vi "USB2XXX_PowerAnalyzer_Test.vi"() -> ()   [LabVIEW 2010]
panel:
  in  "FilterLevel":i32=500
  in  "UseZeroSet":u8=1
  in  "AutoZeroSet":u8
  out "功率":dbl[](graph)=[0.0, 0.0, 0.0, 0.0, 0.0, 0.0, 1.7578661454081409e-07, 0.0, 0.0, 0.0, 0.0, 0.0, 0.0, 0.0, 0.0, 0.0, 0.0, 0.0, 0.0, 0.0, 0.0, 0.0, 0.0, 1.7578661454081409e-07, 0.0, 1.7578661454081409e-07, 0.0, 0.0, 0.0, 0.0]
  out "电压":dbl[](graph)
  out "电流":dbl[](graph)=[0.0, 0.0, 0.0, 0.0, 0.0, 0.0009375143053330281, 0.0, 0.0, 0.0, 0.0, 0.0, 0.0, 0.0009375143053330281, 0.0009375143053330281, 0.0009375143053330281, 0.0, 0.0, 0.0009375143053330281, 0.0009375143053330281, 0.0, 0.0, 0.0, 0.0009375143053330281, 0.0, 0.0, 0.0009375143053330281, 0.0009375143053330281, 0.0, 0.0, 0.0]
  in  "stop":bool
  in  "SamplingRate":i32=1000
  in  "Device Index":i32(ring) items=["0", "1", "2", "3", "4", "5"]
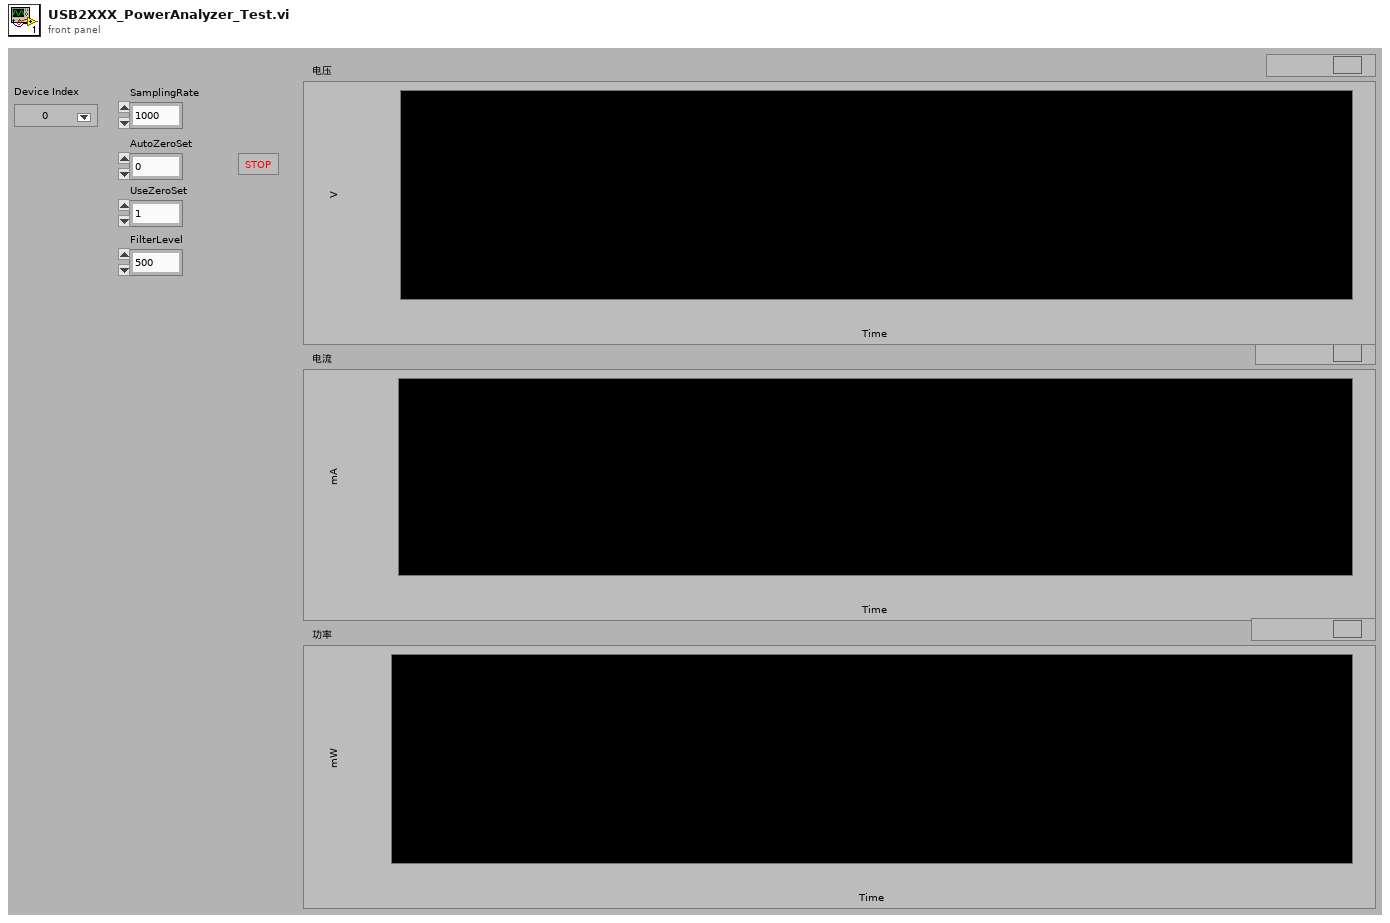
[diagram p1: front panel]
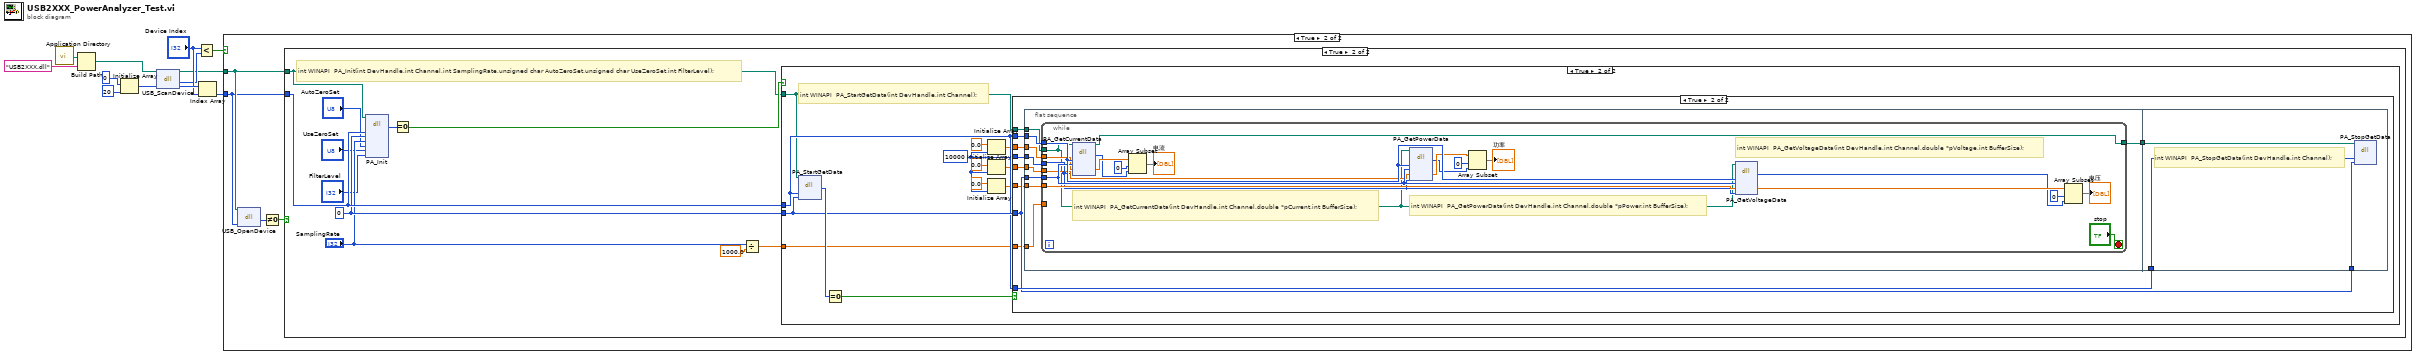
[diagram p0: block diagram]
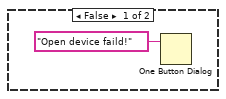
[diagram p3: hidden frame]
diagram:
  n1 = call <vilib>:"Application Directory.vi"() -> ("Application Directory"=w2:path)
  n2 = Build Path(base path=w2, name or relative path="USB2XXX.dll") -> (appended path=w1:path)
  n3 = Initialize Array(0, 20 ("dimension size")) -> (w9:i32[])
  n4 = dll-call lib="E:/OtherWork/STM32/USB2XXX_Example/trunk/Labview/PublicFiles/USB2XXX.dll" fn="USB_ScanDevice"(path in=w1, "pDevNum"=w9) -> (path out=w5:path, "return type"=w7:i32, "pDevNum"=w12:i32[])  [unwired: 2 in, 1 out]
  n5 = Less?(x="Device Index", y=w7) -> (x < y?=w6:bool)
  n6 = Index Array(array=w12, index="Device Index") -> (element=w4:i32)
  n7 = case shown="True" w6 {
    tunnel: w5 -> [_ w14]
    tunnel: w4 -> [_ w13]
    frame False {
    }
    frame True {
      n8 = dll-call lib="E:/OtherWork/STM32/USB2XXX_Example/trunk/Labview/PublicFiles/USB2XXX.dll" fn="USB_OpenDevice"(path in=w14, "DevIndex"=w13) -> ("return type"=w16:u8)  [unwired: 3 in, 2 out]
      n9 = Not Equal To 0?(x=w16) -> (x != 0?=w15:bool)
      n10 = case shown="True" w15 {
        tunnel: w13 -> [_ w24]
        tunnel: w14 -> [_ w25]
        frame False {
          n11 = One Button Dialog(message="Open device faild!") -> ()  [unwired: 1 in, 1 out]
        }
        frame True {
          w23 = 0 ("Channel")
          # "int WINAPI  PA_Init(int DevHandle,int Channel,int SamplingRate,unsigned char AutoZeroSet,unsigned char UseZeroSet,int FilterLevel);"
          n12 = dll-call lib="E:/Projects/USB2XXX/trunk/USB2XXX/USB2XXX/vs2010/Release/USB2XXX.*" fn="PA_Init"(path in=w25, "DevHandle"=w24, "Channel"=w23, "SamplingRate"="SamplingRate", "AutoZeroSet"="AutoZeroSet", "UseZeroSet"="UseZeroSet", "FilterLevel"="FilterLevel") -> ("return type"=w18:i32)  [unwired: 8 in, 2 out]
          n13 = Equal To 0?(x=w18) -> (x = 0?=w28:bool)
          n14 = Divide(x="SamplingRate", y=1000.0 ("element")) -> (x/y=w26:dbl)
          n15 = case shown="True" w28 {
            tunnel: w24 -> [_ w38]
            tunnel: w23 -> [_ w39]
            tunnel: w26 -> [_ w30]
            tunnel: w25 -> [_ w29]
            frame False {
            }
            frame True {
              w31 = 10000 ("dimension size")
              # "int WINAPI  PA_StartGetData(int DevHandle,int Channel);"
              n16 = dll-call lib="E:/Projects/USB2XXX/trunk/USB2XXX/USB2XXX/vs2010/Release/USB2XXX.*" fn="PA_StartGetData"(path in=w29, "DevHandle"=w38, "Channel"=w39) -> ("return type"=w41:i32)  [unwired: 4 in, 2 out]
              n17 = Equal To 0?(x=w41) -> (x = 0?=w40:bool)
              n18 = Initialize Array(0.0 ("element"), w31) -> (w34:dbl[])
              n19 = Initialize Array(0.0 ("element"), w31) -> (w33:dbl[])
              n20 = Initialize Array(0.0 ("element"), w31) -> (w32:dbl[])
              n21 = case shown="True" w40 {
                tunnel: w38 -> [_ w51]
                tunnel: w39 -> [_ w49]
                tunnel: w38 -> [_ w50]
                tunnel: w34 -> [_ w48]
                tunnel: w33 -> [_ w47]
                tunnel: w32 -> [_ w46]
                tunnel: w31 -> [_ w45]
                tunnel: w30 -> [_ w44]
                tunnel: w29 -> [_ w43]
                frame False {
                }
                frame True {
                  n22 = flat-sequence {
                    tunnel: w50 -> [w60]
                    tunnel: w49 -> [w59]
                    tunnel: w48 -> [w58]
                    tunnel: w47 -> [w57]
                    tunnel: w46 -> [w56]
                    tunnel: w45 -> [w55]
                    tunnel: w44 -> [w54]
                    tunnel: w43 -> [w53]
                    tunnel: [w52] -> w42
                    tunnel: w51 -> [w84]
                    tunnel: w49 -> [w83]
                    tunnel: w42 -> [w82]
                    frame #0 {
                      n23 = while {
                        tunnel: w60 -> [w80]
                        tunnel: w59 -> [w79]
                        tunnel: w58 -> [w78]
                        tunnel: w57 -> [w77]
                        tunnel: w56 -> [w76]
                        tunnel: w55 -> [w75]
                        tunnel: w54 -> [_]
                        tunnel: w53 -> [w65]
                        tunnel: [w64] -> w52
                        stop <- "stop" stop-if-true
                        # "int WINAPI  PA_GetVoltageData(int DevHandle,int Channel,double *pVoltage,int BufferSize);"
                        # "int WINAPI  PA_GetPowerData(int DevHandle,int Channel,double *pPower,int BufferSize);"
                        # "int WINAPI  PA_GetCurrentData(int DevHandle,int Channel,double *pCurrent,int BufferSize);"
                        n24 = dll-call lib="E:/Projects/USB2XXX/trunk/USB2XXX/USB2XXX/vs2010/Release/USB2XXX.*" fn="PA_GetCurrentData"(path in=w65, "DevHandle"=w80, "Channel"=w79, "pCurrent"=w78, "BufferSize"=w75) -> (path out=w64:path, "return type"=w72:i32, "pCurrent"=w74:dbl[])  [unwired: 5 in, 1 out]
                        n25 = Array Subset(array=w74, index=0, length=w72) -> (→"电流":dbl[])
                        n26 = dll-call lib="E:/Projects/USB2XXX/trunk/USB2XXX/USB2XXX/vs2010/Release/USB2XXX.*" fn="PA_GetPowerData"(path in=w65, "DevHandle"=w80, "Channel"=w79, "pPower"=w77, "BufferSize"=w75) -> ("return type"=w66:i32, "pPower"=w69:dbl[])  [unwired: 5 in, 2 out]
                        n27 = Array Subset(array=w69, index=0, length=w66) -> (→"功率":dbl[])
                        n28 = dll-call lib="E:/Projects/USB2XXX/trunk/USB2XXX/USB2XXX/vs2010/Release/USB2XXX.*" fn="PA_GetVoltageData"(path in=w65, "DevHandle"=w80, "Channel"=w79, "pVoltage"=w76, "BufferSize"=w75) -> ("return type"=w67:i32, "pVoltage"=w68:dbl[])  [unwired: 5 in, 2 out]
                        n29 = Array Subset(array=w68, index=0, length=w67) -> (→"电压":dbl[])
                      }
                    }
                    frame #1 {
                      # "int WINAPI  PA_StopGetData(int DevHandle,int Channel);"
                      n30 = dll-call lib="E:/Projects/USB2XXX/trunk/USB2XXX/USB2XXX/vs2010/Release/USB2XXX.*" fn="PA_StopGetData"(path in=w82, "DevHandle"=w84, "Channel"=w83) -> ()  [unwired: 5 in, 2 out]
                    }
                  }
                }
              }
            }
          }
        }
      }
    }
  }
